vi "Configure Weights.vi"(7 "Config Manager in":refnum<class "Config Manager Class.lvclass">, 8 "error in":errorcluster, 11 "WorkTable in":refnum<class "WorkTable Class.lvclass">) -> (0 "error out":errorcluster, 3 "WorkTable out":refnum<class "WorkTable Class.lvclass">)   [LabVIEW 2011, in "WorkTable Class.lvclass"]
uses:
  WorkTable Class.lvclass
  Config Manager Class/Config Manager Class.lvclass
  Type Definitions/Worktable_Weights.ctl
  Utils/Type Definitions/Position_Orientation.ctl
  Vec3d Class/Vec3d Class.lvclass
  Orient3d Class/Orient3d Class.lvclass
  Config Manager Class/Type Definitions/Manifold Channel Types.ctl
  Config Manager Class/Type Definitions/Part Type.ctl
  Config Manager Class/Read Manifold Channel Other.vi
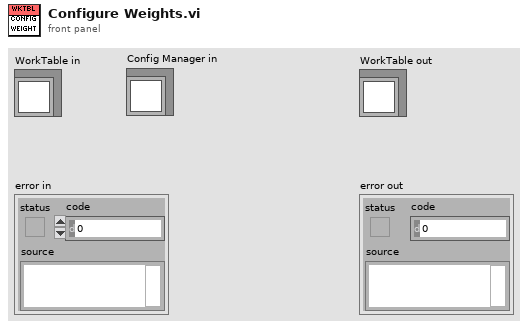
[diagram p1: front panel]
types:
  T1 = typedef "Worktable_Weights.ctl" = cluster{"Weight Slots":cluster{"Weight State":enum16{"Empty", "Populated"}, "Weight Type":enum16{"Weight 1", "Weight 2", "Weight 3", "Weight 4"}, "Location/Orientation":T2}[], "Vacuum Channel":i32}
  T2 = typedef "Position_Orientation.ctl" = cluster{"Center":refnum<class "Vec3d Class.lvclass">, "Orientation":refnum<class "Orient3d Class.lvclass">}
  T3 = typedef "Manifold Channel Types.ctl" = enum16{"GANTRY_HEAD_OUTER", "GANTRY_HEAD_INNER", "GLUE_RESERVOIR_CHUCK", "STAMP_TOOL_CHUCK", "WEIGHT_TOOL_CHUCK"}
  T4 = enum16{"Weight 1", "Weight 2", "Weight 3", "Weight 4"}
  T5 = cluster{"Weight State":enum16{"Empty", "Populated"}, "Weight Type":enum16{"Weight 1", "Weight 2", "Weight 3", "Weight 4"}, "Location/Orientation":T2}
  T6 = typedef "Part Type.ctl" = enum16{"BBM", "HDI", "GLUERESERVOIR", "STAMP", "WEIGHT"}
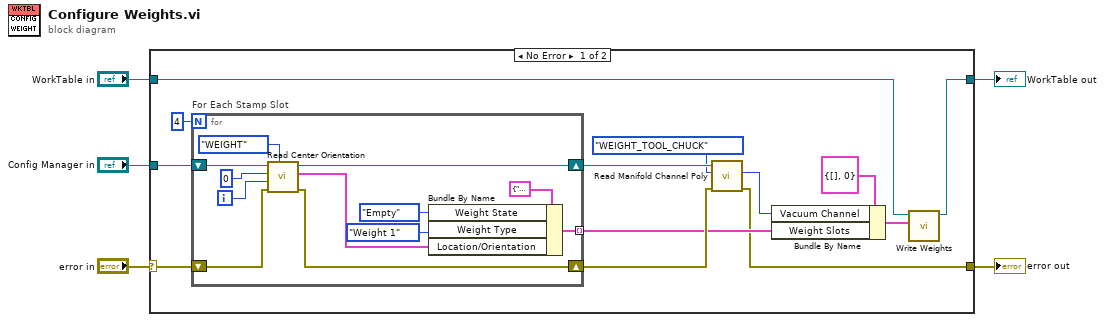
[diagram p0: block diagram]
diagram:
  n1 = case shown="No Error" "error in" {
    selector: "error in" -> [w14 w32]
    tunnel: [w8 w32] -> w1
    tunnel: [w17 w31] -> w2
    tunnel: "WorkTable in" -> [w18 w31]
    tunnel: "Config Manager in" -> [w15 _]
    frame No Error {
      n2 = for "For Each Stamp Slot" {
        N: 4 ("dimension size") -> [_]
        tunnel: [w30] -> w10 mode=indexing
        shift-right: [w23] -> w11
        shift-left: w14 -> [w27]
        shift-right: [w22] -> w13
        shift-left: w15 -> [w29]
        i -> [w25]
        n3 = call "Read Center Orientation.vi"("Part Type"=Part_Type."WEIGHT", "error in"=w27, "slot"=w25, "chuck"=0, "Config Manager in"=w29) -> ("error out"=w23:errorcluster, "Location/Orientation"=w24:T2, "Config Manager out"=w22:refnum<class "Config Manager Class.lvclass">)  [unwired: 4 in]
        n4 = Bundle By Name(cluster=T5 {"Weight State"=enum."Empty", "Weight Type"=enum."Weight 1", "Location/Orientation"={"Center"=refnum, "Orientation"=refnum}} ("element"), "Weight State"=enum16{"Empty", "Populated"}."Empty", "Weight Type"=T4."Weight 1", "Location/Orientation"=w24) -> (w30:T5)
      }
      n5 = call-poly "Read Manifold Channel Poly.vi"("error in"=w11, "Manifold Channel Type"=Manifold_Channel_Types."WEIGHT_TOOL_CHUCK", "Config Manager in"=w13) -> ("error out"=w8:errorcluster, "Channel"=w9:i32)  [unwired: 6 in, 1 out]
      n6 = Bundle By Name(cluster=T1 {"Weight Slots"=[], "Vacuum Channel"=0} ("Weights"), "Vacuum Channel"=w9, "Weight Slots"=w10) -> (w6:T1)
      n7 = call-dynamic "Write Weights.vi"("Weights"=w6, "WorkTable Class in"=w18) -> ("WorkTable Class out"=w17:refnum<class "WorkTable Class.lvclass">)  [unwired: 8 in, 1 out]
    }
    frame Error {
    }
  }
  "WorkTable out" <- w2
  "error out" <- w1
